vi "assign FPGA resources from Server to Client.vi"(8 "error in (no error)":errorcluster, 11 "Device Item Ref in":T1 format="%.0x") -> (0 "error out":errorcluster, 3 "Device Item Ref out":T1 format="%.0x")   [LabVIEW 2016, in "FPGA RM System Definition API.lvlib"]
doc: "Use this VI in the FPGA Addon's ActionVIOnCompile to assign FPGA resources to another custom device in the System Definition"
uses:
  FPGA RM System Definition API.lvlib
  <vilib>/NI Veristand/Custom Device API/Custom Device Item Ref.ctl
  Shared/FG Action.ctl
  Shared/FPGA Configuration Classes/FPGA Device/FPGA Device.lvclass
  Shared/FPGA Configuration Classes/FPGA Device/FPGA Device.lvclass/FPGA Device.ctl
  Shared/FPGA Configuration Classes/FPGA Device/Write RIO Device Name.vi
  Shared/FPGA Configuration Classes/FPGA Device/Write bitfile path.vi
  <vilib>/NI Veristand/Custom Device API/NI VeriStand - Get Item Property.vi
  <vilib>/NI Veristand/Custom Device API/Get Item Property (Path).vi
  <vilib>/NI Veristand/Custom Device API/Get Item Property (String).vi
  <vilib>/NI Veristand/Custom Device API/NI VeriStand - Set Item Property.vi
  <vilib>/NI Veristand/Custom Device API/Set Item Property (Path).vi
  <vilib>/NI Veristand/Custom Device API/Set Item Property (String).vi
  Shared/FPGA RM Shared API.lvlib
  Shared/FPGA Configuration Classes/Channel Group/Channel group.lvclass
  Shared/FPGA Configuration Classes/Datatype Group/Datatype group.lvclass
  <vilib>/NI VeriStand/Custom Device API/Custom Device API.lvlib
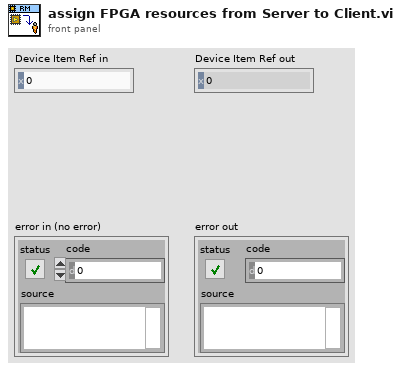
[diagram p1: front panel]
types:
  T1 = typedef "Custom Device API.lvlib/Custom Device Item Ref.ctl" = u64
  T2 = typedef "FPGA RM Shared API.lvlib/FG Action.ctl" = enum8{"GET", "SET"}
  T3 = typedef "FPGA RM Shared API.lvlib/fpga resource.ctl" = cluster{"name":string, "datatype":string, "channel type":T4, "value":variant, "notes":string}
  T4 = typedef "FPGA RM Shared API.lvlib/Channel Type.ctl" = enum16{"Write Channel", "Read Channel", "Write Waveform", "Read Waveform"}
  T5 = typedef "FPGA RM Shared API.lvlib/FPGA Settings.ctl" = cluster{"Bitfile path":path, "RIO Device Address":string}
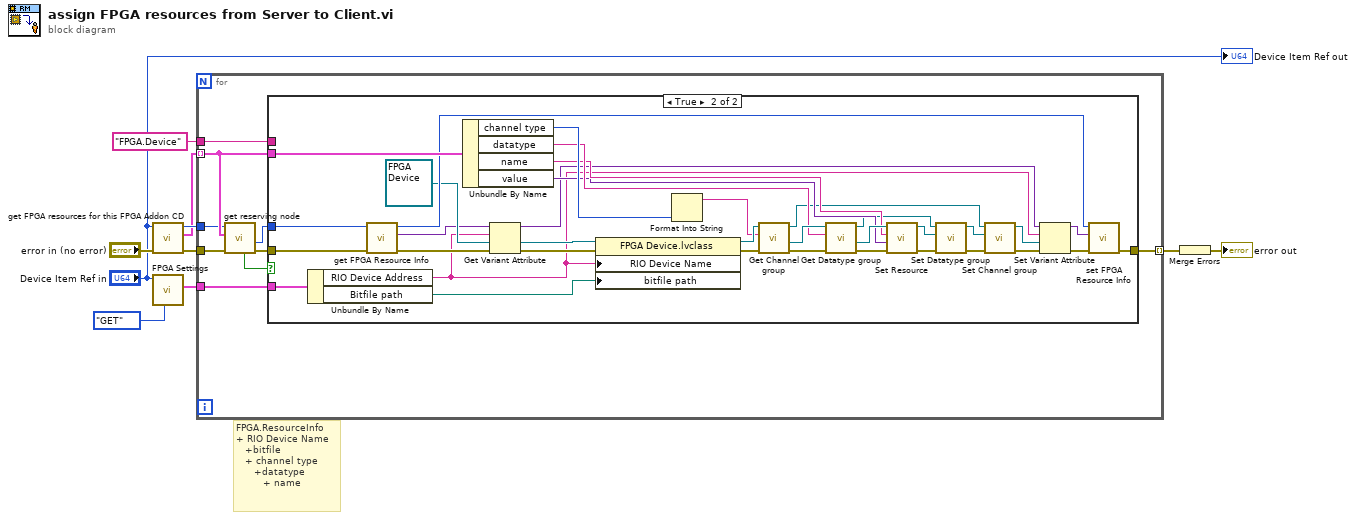
[diagram p0: block diagram]
diagram:
  # "FPGA.ResourceInfo\n+ RIO Device Name\n   +bitfile\n   + channel type\n      +datatype\n         + name"
  n1 = call "get FPGA resources for this FPGA Addon CD.vi"("error in (no error)"="error in (no error)", "Item Ref in"="Device Item Ref in") -> ("error out"=w10:errorcluster, "fpga resources"=w7:T3[], "Item Ref out"=w8:T1)  [unwired: 6 in, 1 out]
  n2 = call "FPGA Settings.vi"("Action"=FG_Action."GET", "Item Ref"="Device Item Ref in") -> ("FPGA Settings"=w3:T5)  [unwired: 7 in, 2 out]
  n3 = for {
    tunnel: w7 -> [w19] mode=indexing
    tunnel: w8 -> [w14]
    tunnel: w10 -> [w18]
    tunnel: [w16] -> w6 mode=indexing
    tunnel: "FPGA.Device" ("FPGA.Device") -> [w13]
    tunnel: w3 -> [w11]
    n4 = call "get reserving node.vi"("error in (no error)"=w18, "FPGA Resource"=w19, "Item Ref in"=w14) -> ("error out"=w15:errorcluster, "Dependent Node Ref"=w17:T1, "Found"=w12:bool)  [unwired: 5 in, 1 out]
    n5 = case shown="True" w12 {
      tunnel: w19 -> [_ w55]
      tunnel: w17 -> [_ w51]
      tunnel: [w20 w54] -> w16
      tunnel: w15 -> [w20 w53]
      tunnel: w13 -> [_ _]
      tunnel: w11 -> [_ w49]
      frame False {
      }
      frame True {
        n6 = Unbundle By Name(w49) -> ("RIO Device Address"=w21:string, "Bitfile path"=w48:path)
        n7 = call "get FPGA Resource Info.vi"("error in (no error)"=w53, "CD Ref in"=w51) -> ("error out"=w30:errorcluster, "Value"=w34:variant, "Item Ref out"=w50:T1)  [unwired: 7 in]
        n8 = Unbundle By Name(w55) -> ("channel type"=w52:T4, "datatype"=w44:string, "name"=w42:string, "value"=w41:variant)
        n9 = Get Variant Attribute(Variant=w34, name=w21, default value (empty Variant)=refnum<class "FPGA Device.lvclass"> refnum ("FPGA RM Shared API.lvlib:FPGA Device.lvclass"), error in=w30) -> (duplicate Variant=w32:variant, value=w35:refnum<class "FPGA Device.lvclass">, error out=w29:errorcluster)  [unwired: 1 out]
        n10 = property class="FPGA Device.lvclass"(reference=w35, error in=w29, "RIO Device Name"=w21, "bitfile path"=w48) -> (reference out=w47:refnum<class "FPGA Device.lvclass">, error out=w28:errorcluster)
        n11 = Format Into String(w52) -> (resulting string=w46:string)  [unwired: 3 in, 1 out]
        n12 = call "Get Channel group.vi"("error in (no error)"=w28, "name"=w46, "FPGA Device in"=w47) -> ("error out"=w27:errorcluster, "Datatype group"=w45:refnum<class "Channel group.lvclass">, "FPGA Device out"=w38:refnum<class "FPGA Device.lvclass">)  [unwired: 5 in, 1 out]
        n13 = call "Get Datatype group.vi"("error in (no error)"=w27, "name"=w44, "Channel group in"=w45) -> ("error out"=w26:errorcluster, "Datatype group"=w43:refnum<class "Datatype group.lvclass">, "Channel group out"=w39:refnum<class "Channel group.lvclass">)  [unwired: 5 in, 1 out]
        n14 = call "Set Resource.vi"("error in (no error)"=w26, "resource info"=w41, "name in bitfile"=w42, "Datatype group in"=w43) -> ("error out"=w25:errorcluster, "Datatype group out"=w40:refnum<class "Datatype group.lvclass">)  [unwired: 5 in, 1 out]
        n15 = call "Set Datatype group.vi"("error in (no error)"=w25, "Datatype group in"=w40, "Channel group in"=w39) -> ("error out"=w24:errorcluster, "Channel group out"=w37:refnum<class "Channel group.lvclass">)  [unwired: 6 in, 1 out]
        n16 = call "Set Channel group.vi"("error in (no error)"=w24, "Channel group in"=w37, "FPGA Device in"=w38) -> ("error out"=w23:errorcluster, "FPGA Device out"=w33:refnum<class "FPGA Device.lvclass">)  [unwired: 6 in, 1 out]
        n17 = Set Variant Attribute(Variant=w32, name=w21, value=w33, error in=w23) -> (Variant out=w31:variant, error out=w22:errorcluster)  [unwired: 1 out]
        n18 = call "set FPGA Resource Info.vi"("error in (no error)"=w22, "Value"=w31, "Relative Item Ref Out"=w50) -> ("error out"=w54:errorcluster)  [unwired: 7 in, 1 out]
      }
    }
  }
  n19 = Merge Errors(w6) -> (→"error out":errorcluster)
  "Device Item Ref out" <- "Device Item Ref in"
